vi "Filter Class Tree by Type.vi"(10 "Show":T1, 11 "Class Tree Array":T2(array[cluster])) -> (3 "Class Tree Array":T2(array[cluster]))   [LabVIEW 2023]
panel:
  out "Numeric":i32
  # "To maintain tree indents, we must retain all parents (as disabled) if they don't match the filter, or else the tree item inset will break"
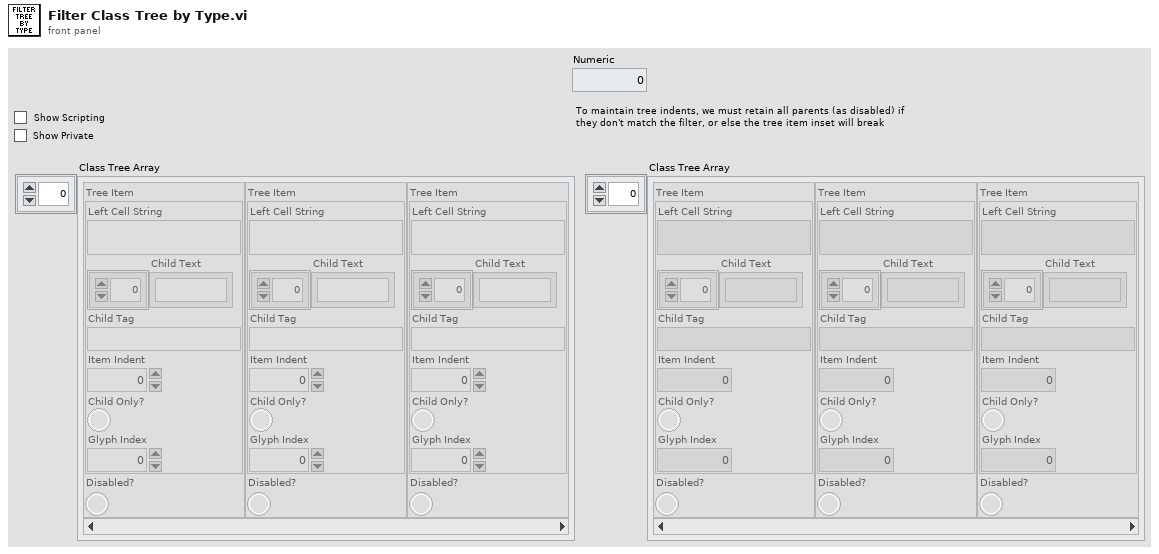
[diagram p1: front panel]
types:
  T1 = cluster{"Show Scripting":bool, "Show Private":bool}
  T2 = cluster{"Tree Item":cluster{"Left Cell String":string, "Child Text":string[], "Child Tag":string, "Item Indent":i32, "Child Only?":bool, "Glyph Index":i32}, "Disabled?":bool}[]
  T3 = cluster{"Index":u16, "Property Type":enum16{"Unknown", "Base", "Scripting", "Private", "Deprecated", "None", "Divider"}, "ID String":string, "Dotted ID String":string, "Class":string, "Parent":string, "Display name full":string, "Display name short":string, "Parents Array":string[], "Indent":u16}
  T4 = cluster{"Tree Item":cluster{"Left Cell String":string, "Child Text":string[], "Child Tag":string, "Item Indent":i32, "Child Only?":bool, "Glyph Index":i32}, "Disabled?":bool}
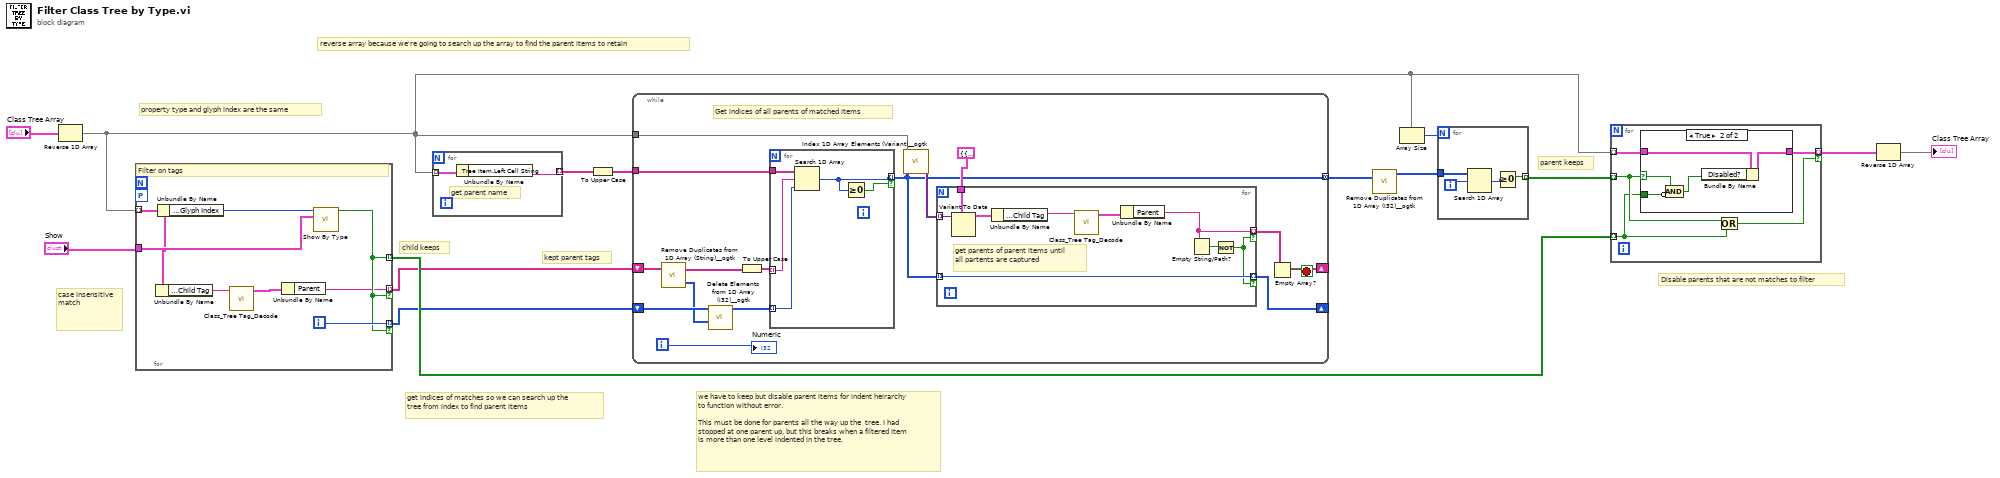
[diagram p0: block diagram]
diagram:
  # "property type and glyph index are the same"
  # "get indices of matches so we can search up the tree from index to find parent items"
  # "reverse array because we're going to search up the array to find the parent items to retain"
  # "Disable parents that are not matches to filter"
  # "parent keeps"
  # "we have to keep but disable parent items for indent heirarchy to function without error.\n\nThis must be done for parents all the way up the  tree. I had stopped at one parent up, but this breaks when a filtered item is more than one level indented in the tree."
  # "kept parent tags"
  # "child keeps"
  # "case insensitive match"
  n1 = Reverse 1D Array(array="Class Tree Array") -> (reversed array=w6:T2)
  n2 = for {
    tunnel: "Show" -> [w22]
    workers-P: _ -> [_]
    tunnel: w6 -> [w17] mode=indexing
    tunnel: [w20] -> w11 mode=indexing
    tunnel: [w18] -> w4 mode=indexing if=w20
    tunnel: [w21] -> w3 mode=indexing if=w20
    i -> [w21]
    # "Filter on tags"
    n3 = Unbundle By Name(w17) -> ("Tree Item.Child Tag"=w16:string)
    n4 = Unbundle By Name(w17) -> ("Tree Item.Glyph Index"=w19:i32)
    n5 = call "Class_Tree Tag_Decode.vi"("Tag In"=w16) -> ("TagData"=w15:T3)  [unwired: 10 in]
    n6 = Unbundle By Name(w15) -> ("Parent"=w18:string)
    n7 = call "Show By Type.vi"("Show"=w22, "Item's Property Type"=w19) -> ("Show"=w20:bool)  [unwired: 9 in]
  }
  n8 = for {
    tunnel: w6 -> [w24] mode=indexing
    tunnel: [w23] -> w12 mode=indexing
    # "get parent name"
    n9 = Unbundle By Name(w24) -> ("Tree Item.Left Cell String"=w23:string)
  }
  n10 = To Upper Case(1:w12) -> (0:w5:string[])
  n11 = while {
    tunnel: w6 -> [w37]
    shift-right: [w35] -> _
    shift-left: w4 -> [w29]
    tunnel: [w31] -> w2 mode=concatenating
    tunnel: w5 -> [w38]
    shift-right: [w30] -> _
    shift-left: w3 -> [w28]
    i -> [w34]
    stop <- w39 stop-if-true
    # "Get indices of all parents of matched items"
    n12 = call <userlib>:"Remove Duplicates from 1D Array (String)__ogtk.vi"("Input Array"=w29) -> ("Output Array"=w25:string[], "indices of removed elements"=w27:i32[])
    n13 = call <userlib>:"Delete Elements from 1D Array (I32)__ogtk.vi"("indices"=w27, "array"=w28) -> ("array w/ subset deleted"=w26:i32[])  [unwired: 8 in, 1 out]
    n14 = To Upper Case(1:w25) -> (0:w32:string[])
    n15 = for {
      tunnel: w32 -> [w51] mode=indexing
      tunnel: [w50] -> w31 mode=indexing if=w53
      tunnel: w38 -> [w52]
      tunnel: w26 -> [w49] mode=indexing
      n16 = Search 1D Array(1D array=w52, element=w51, start index (0)=w49) -> (index of element=w50:i32)
      n17 = Greater Or Equal To 0?(x=w50) -> (x >= 0?=w53:bool)
    }
    n18 = call <userlib>:"Index 1D Array Elements (Variant)__ogtk.vi"("indices"=w31, "array"=w37) -> ("elements"=w36:variant[])  [unwired: 9 in]
    n19 = for {
      tunnel: w36 -> [w48] mode=indexing
      tunnel: [w42] -> w35 mode=indexing if=w44
      tunnel: [w46] -> w30 mode=indexing if=w44
      tunnel: w31 -> [w46] mode=indexing
      tunnel: T4 {"Tree Item"={"Left Cell String"="", "Child Text"=[], "Child Tag"="", "Item Indent"=0, "Child Only?"=FALSE, "Glyph Index"=0}, "Disabled?"=FALSE} ("Property For Tree with Disabled") -> [w43]
      # "get parents of parent items until all partents are captured"
      n20 = Variant To Data(type=w43, Variant=w48) -> (data=w47:T4)  [unwired: 1 in, 1 out]
      n21 = Unbundle By Name(w47) -> ("Tree Item.Child Tag"=w41:string)
      n22 = call "Class_Tree Tag_Decode.vi"("Tag In"=w41) -> ("TagData"=w40:T3)  [unwired: 10 in]
      n23 = Unbundle By Name(w40) -> ("Parent"=w42:string)
      n24 = Empty String/Path?(string/path=w42) -> (empty?=w45:bool)
      n25 = Not(x=w45) -> (.not. x?=w44:bool)
    }
    n26 = Empty Array?(array=w35) -> (empty?=w39:bool)
    "Numeric" <- w34
  }
  n27 = call <userlib>:"Remove Duplicates from 1D Array (I32)__ogtk.vi"("Input Array"=w2) -> ("Output Array"=w1:i32[])  [unwired: 1 out]
  n28 = Array Size(array=w6) -> (size(s)=w14:i32)
  n29 = for {
    N: w14 -> [_]
    tunnel: w1 -> [w57]
    tunnel: [w54] -> w10 mode=indexing
    i -> [w56]
    n30 = Search 1D Array(1D array=w57, element=w56) -> (index of element=w55:i32)  [unwired: 1 in]
    n31 = Greater Or Equal To 0?(x=w55) -> (x >= 0?=w54:bool)
  }
  n32 = for {
    tunnel: [w61] -> w9 mode=indexing if=w59
    tunnel: w6 -> [w62] mode=indexing
    tunnel: w11 -> [w58] mode=indexing
    tunnel: w10 -> [w60] mode=indexing
    n33 = case shown="True" w60 {
      selector: w60 -> [_ w65]
      tunnel: w62 -> [w63 w68]
      tunnel: [w63 w67] -> w61
      tunnel: w58 -> [_ w66]
      frame False {
      }
      frame True {
        n34 = Compound Arithmetic op=AND(w65, invert w66) -> (w64:bool)
        n35 = Bundle By Name(cluster=w68, "Disabled?"=w64) -> (w67:T4)
      }
    }
    n36 = Or(x=w60, y=w58) -> (x .or. y?=w59:bool)
  }
  n37 = Reverse 1D Array(array=w9) -> (reversed array=→"Class Tree Array":T2)
